vi "数据查询筛选弹框.vi"(8 "error in (no error)":errorcluster caption="错误输入（无错误）", 9 "是否初始化":enum16{"init", "keep"}(ring), 10 "database":string="database1.mdb", 11 "table":string(combo)="CODMn") -> (0 "error out":errorcluster caption="错误输出", 1 "确定输出":bool, 2 "显示项":string[](array[string]), 3 "condition":string)   [LabVIEW 2016]
uses:
  <vilib>/addons/database/Auxilliary.llb/DB Tools DataTypes.ctl
  <vilib>/Utility/miscctls.llb/LVPointTypeDef.ctl
  <vilib>/Utility/sysdir.llb/System Directory Type.ctl
  <vilib>/addons/database/Connection.llb/DB Tools Open Connec (String).vi
  <vilib>/addons/database/Connection.llb/Conn Execute.vi
  <vilib>/addons/database/Recordset.llb/Rec Fetch Recordset Data (R).vi
  <vilib>/addons/database/Recordset.llb/Rec Destroy - Connection.vi
  <userlib>/_OpenG.lib/array/array.llb/Remove Duplicates from 1D Array (String)__ogtk.vi
  <vilib>/addons/database/_DB Variant To Data/Database Variant To Data.xnode
  <vilib>/addons/database/NI_Database_API.lvlib
panel:
  in  "实时分钟小时数据":enum32{"实时数据", "分钟数据", "小时数据"}(radio)
  in  "确定":bool
  out "自定义2single":cluster{"起始范围":string, "截止范围":string}
  out "自定义1single":cluster{"起始范围":string, "截止范围":string}
  out "自定义2筛选条件":string[](array[string])
  out "自定义1筛选条件":string[](array[string])
  in  "标签 2":string="从：\n\n\n至："
  in  "自定义数值结束 2":dbl
  in  "自定义数值起始 2":dbl
  in  "自定义结束时间 2":timestamp
  in  "自定义起始时间 2":timestamp
  in  "自定义 2":T1 caption="自定义"
  in  "组合框 2":string(combo)
  in  "标签":string="从：\n\n\n至："
  in  "自定义数值结束":dbl
  in  "自定义数值起始":dbl
  in  "自定义结束时间":timestamp
  in  "自定义起始时间":timestamp
  in  "自定义":T1
  in  "组合框":string(combo)
  out "type":T2[](array[typedef])
  out "所有测量模式":string[](array[string])
  out "数组":string[](array[string])
  out "columns":string[](array[string])
  in  "测量模式":T3
  in  "退出":bool
  in  "清空":bool
  in  "时间标识输入1":T4 format="%<%Y/%m/%d %H:%M:%S>T"
  in  "时间标识输入2":T4 format="%<%Y/%m/%d %H:%M:%S>T"
  # "实时/分钟/小时数据"
  # "日期"
  # "从："
  # "至："
  # "自定义筛选2"
  # "自定义筛选1"
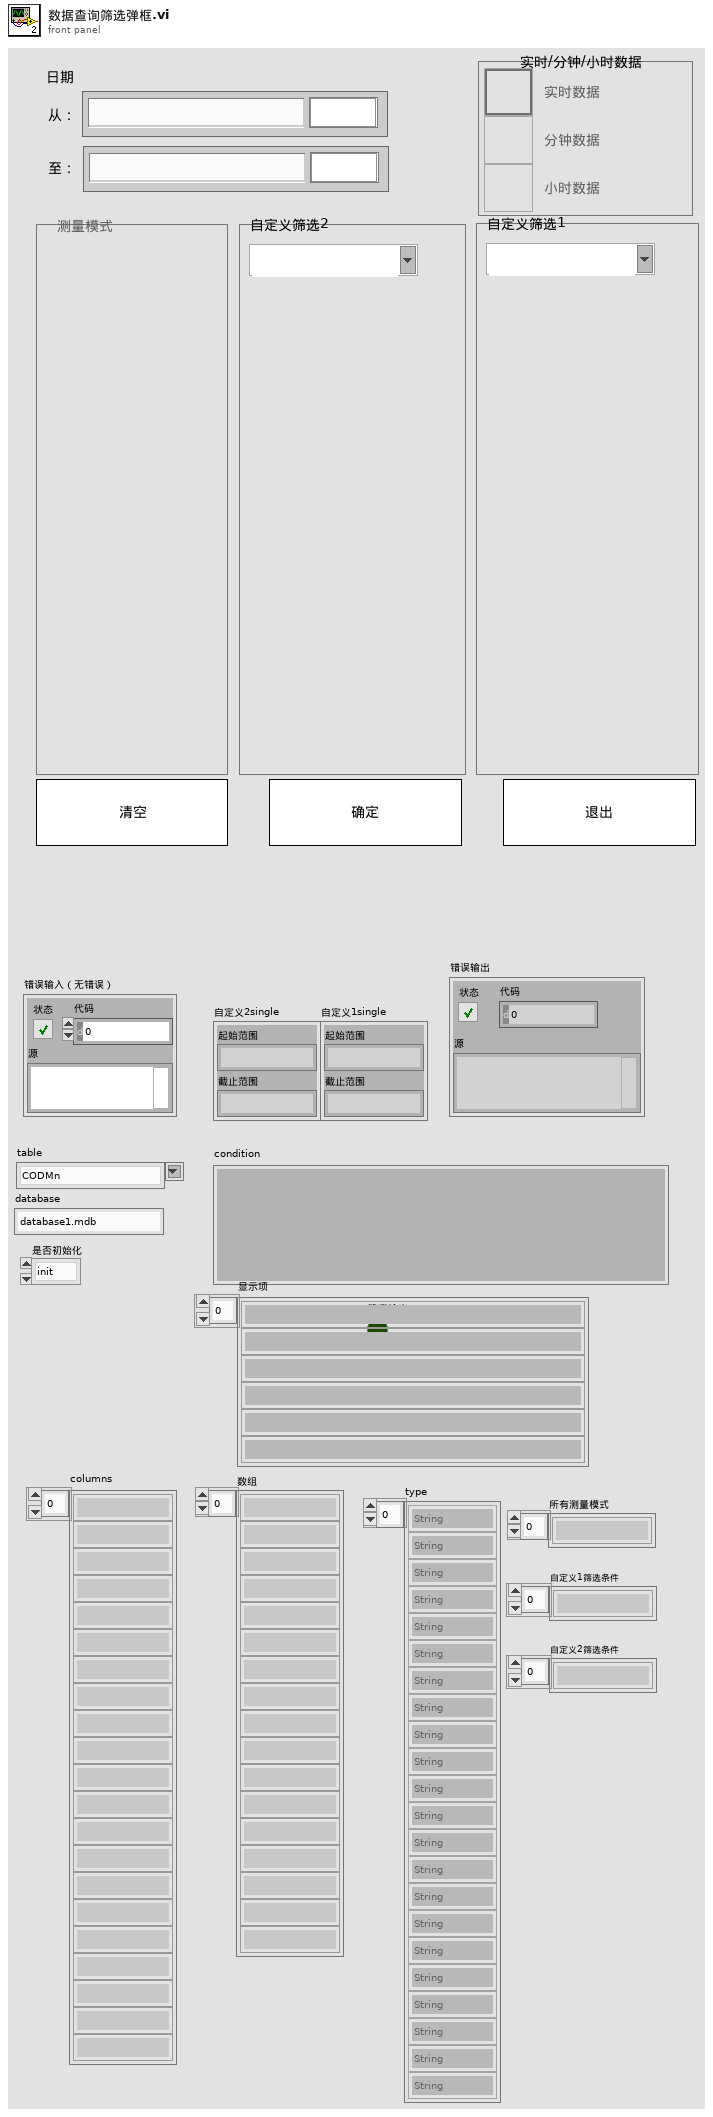
[diagram p1: front panel]
types:
  T1 = cluster{"DSADSA ":bool, "2":bool, "3":bool, "4":bool, "5":bool, "6":bool, "7":bool, "8":bool, "9":bool, "10":bool}
  T2 = typedef "NI_Database_API.lvlib/DB Tools DataTypes.ctl" = enum16{"String", "Long (I32)", "Single (SGL)", "Double (DBL)", "Date/Time", "Binary"}
  T3 = cluster{"水样测试":bool, "标样核查":bool, "零点核查":bool, "跨度核查":bool, "空白测试":bool, "平行样测试":bool, "加标回收":bool, "空白校准":bool, "标样校准":bool, "初始化清洗":bool}
  T4 = typedef "时间标识输入.ctl" = timestamp
  T5 = enum8{"Enabled", "Disabled", "Disabled and Grayed Out"}
  T6 = typedef "LVPointTypeDef.ctl" = cluster{"Horizontal":i16, "Vertical":i16}
  T7 = typedef "System Directory Type.ctl" = i32
  T8 = typedef "NI_Database_API.lvlib/Conn ObjectReference.ctl" = refnum<k1>
  T9 = cluster{"name":string, "database data type":T2, "defined size":i32}[]
  T10 = typedef "NI_Database_API.lvlib/Rec ObjectReference.ctl" = refnum<k1>
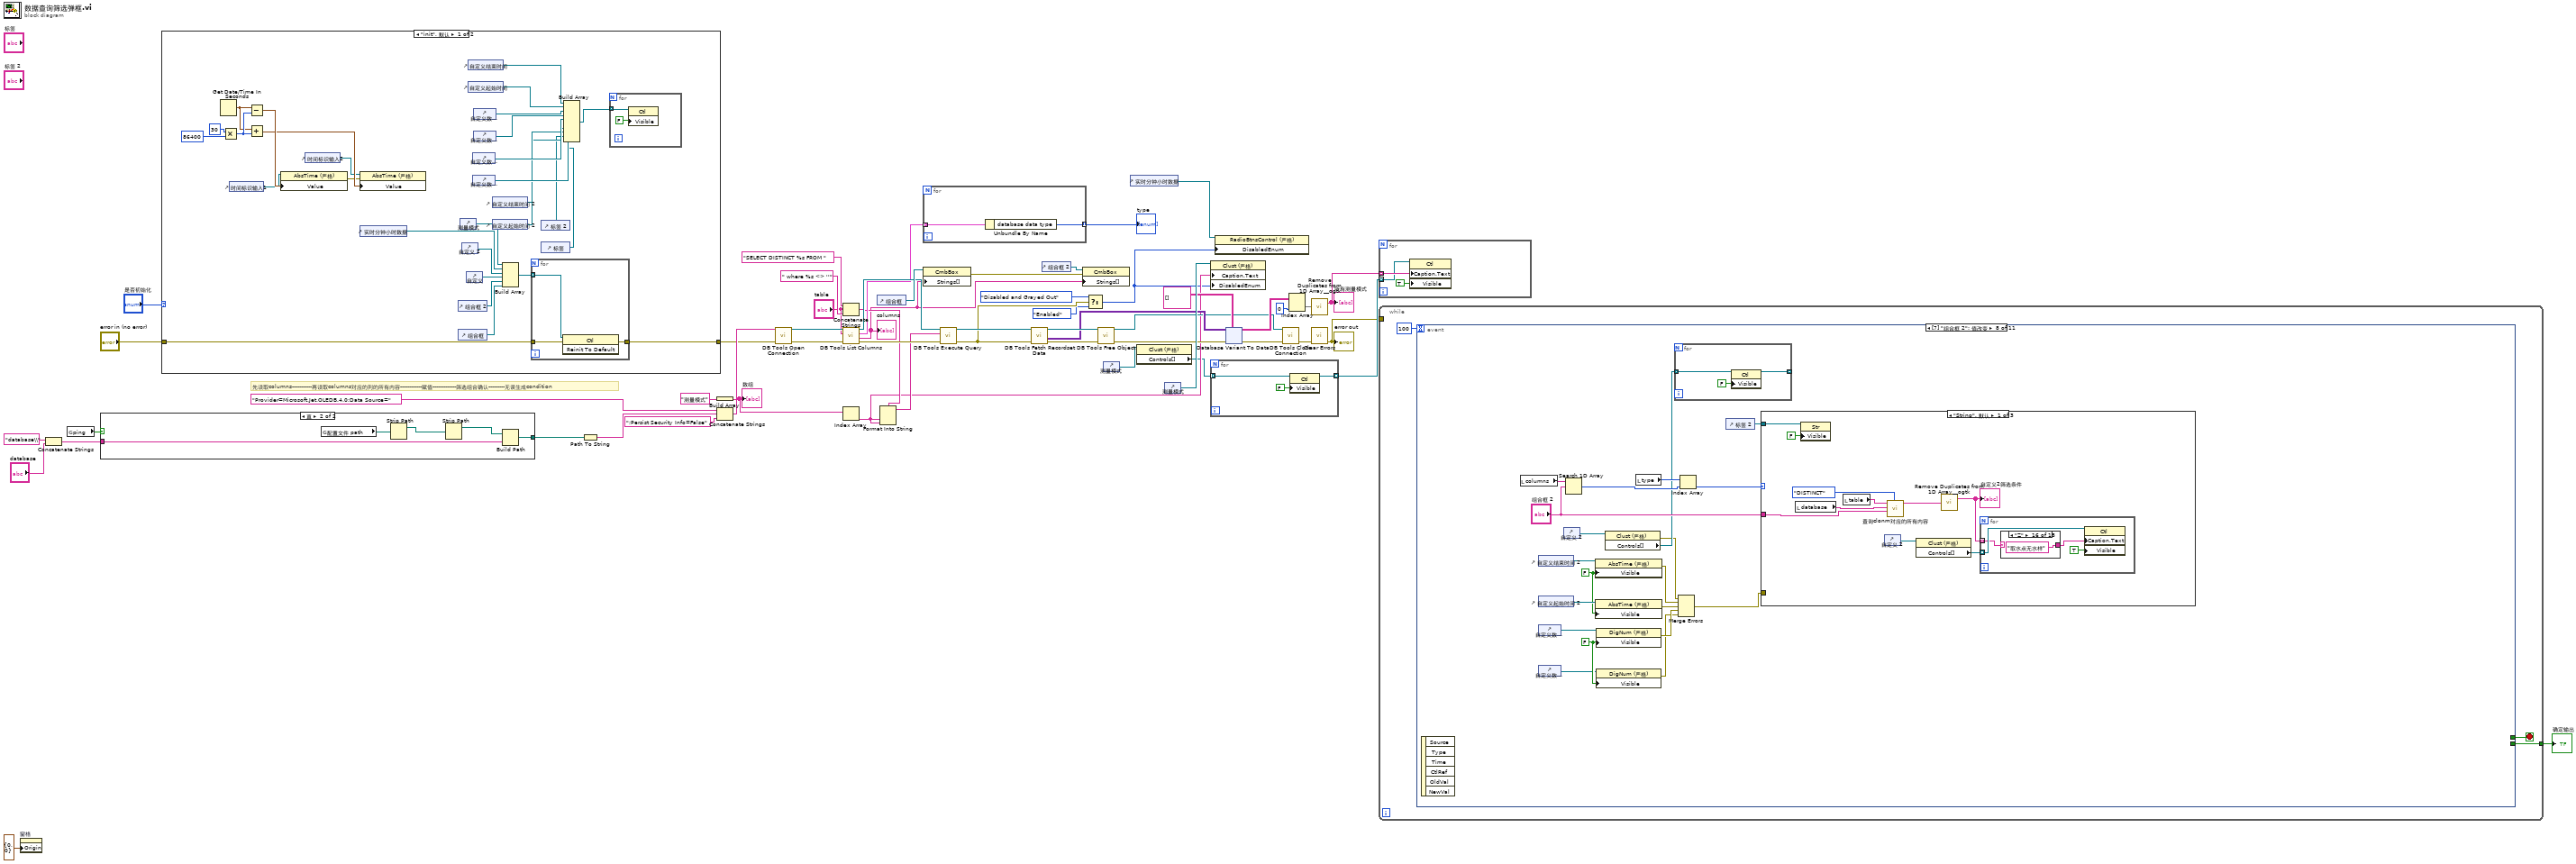
[diagram p0: block diagram]
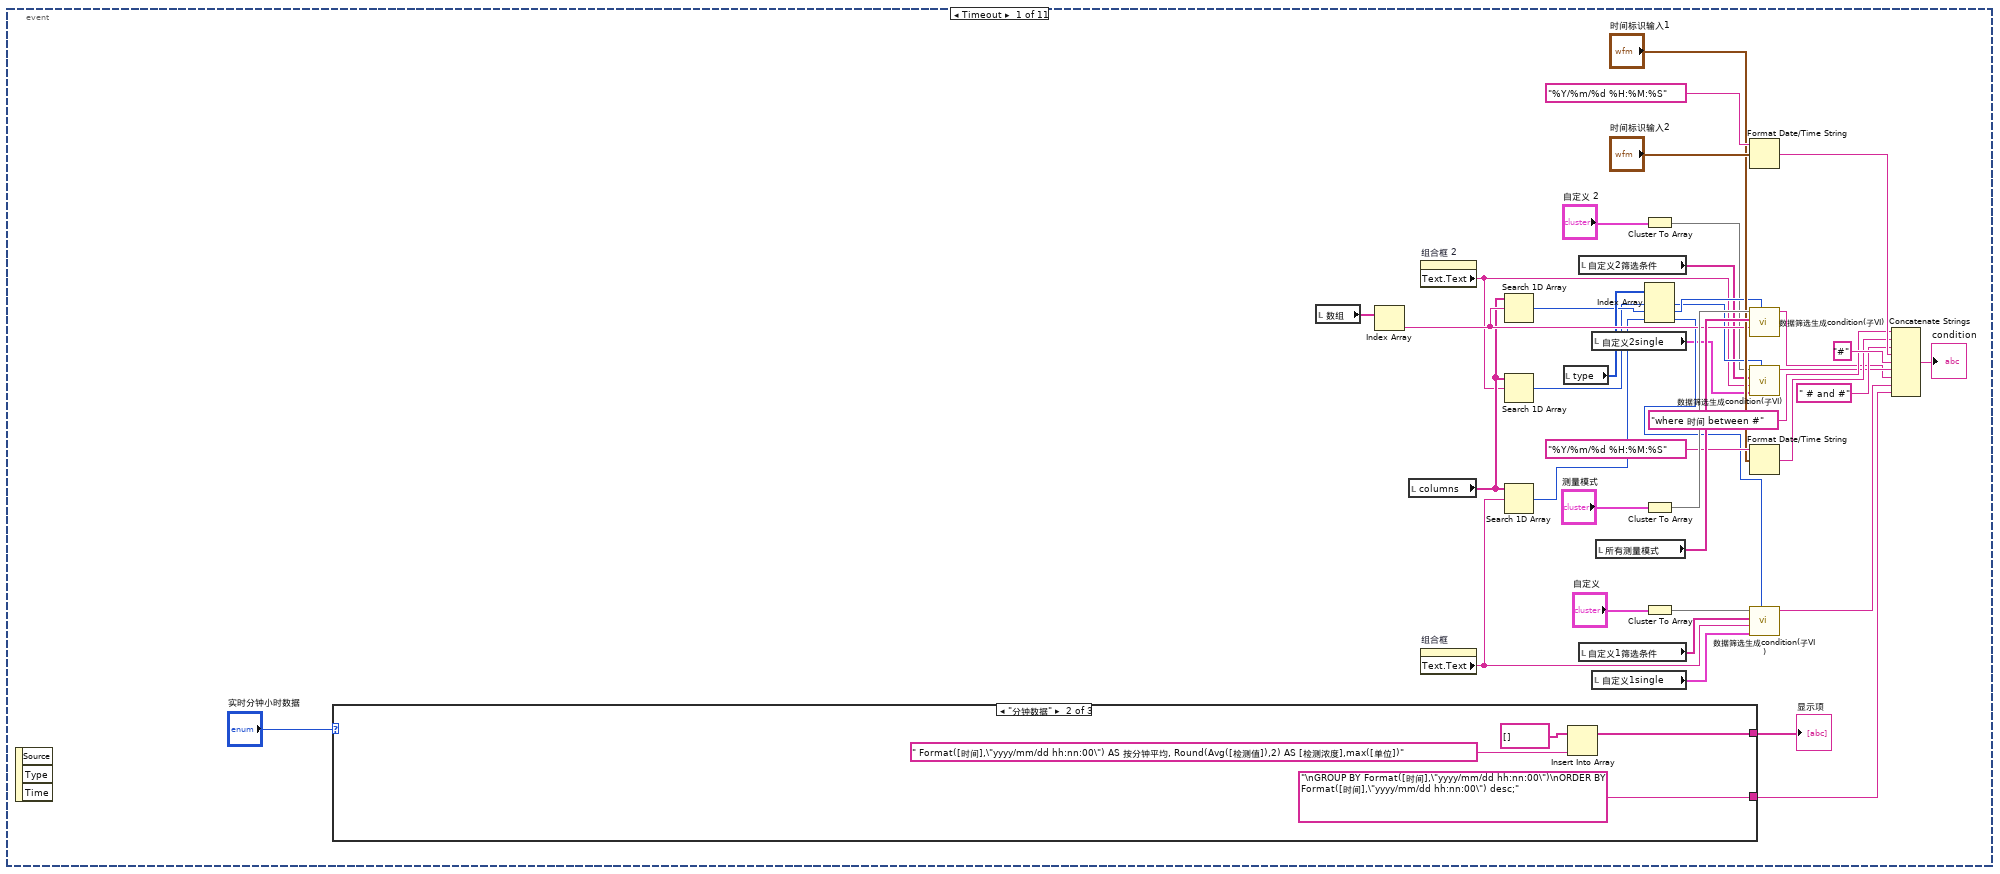
[diagram p3: hidden frame]
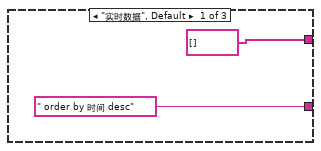
[diagram p4: hidden frame]
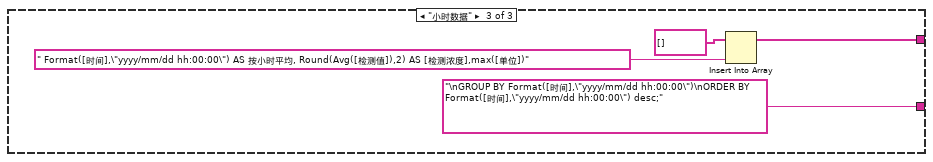
[diagram p5: hidden frame]
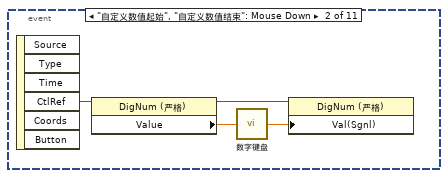
[diagram p6: hidden frame]
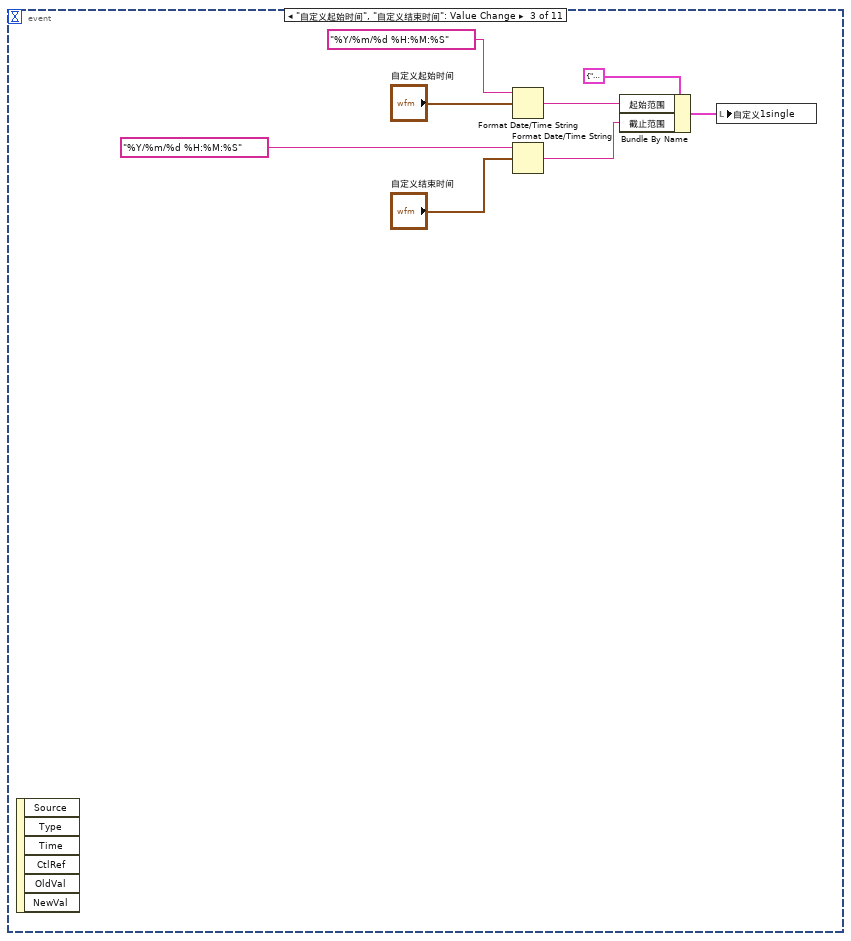
[diagram p7: hidden frame]
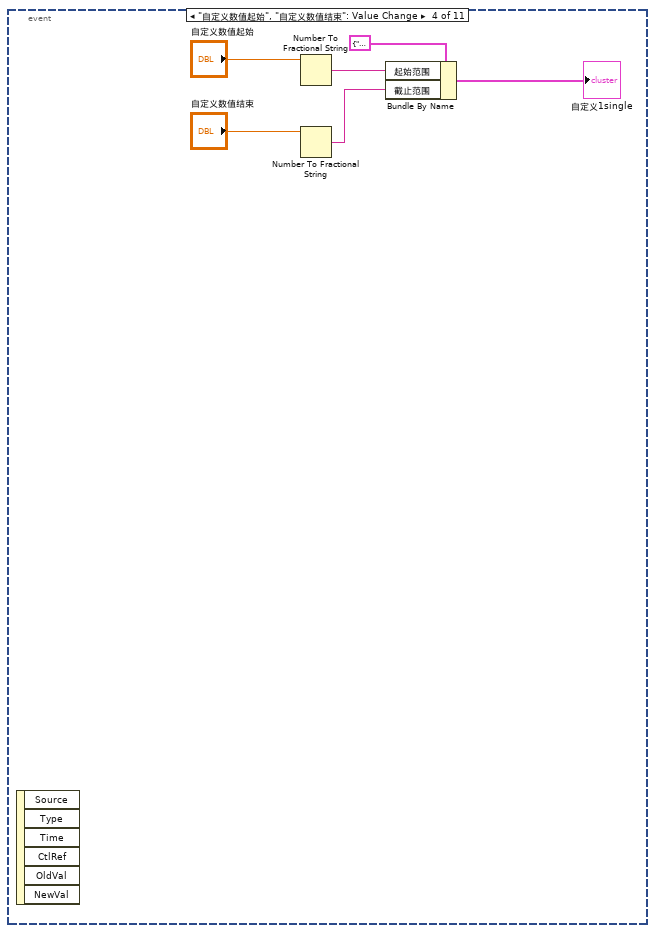
[diagram p8: hidden frame]
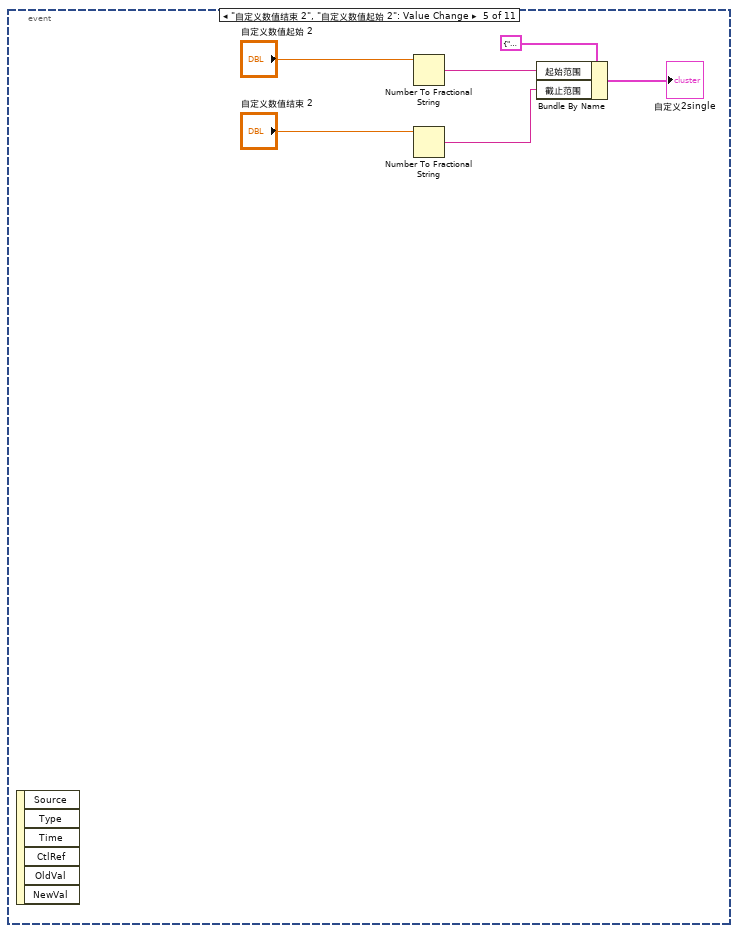
[diagram p9: hidden frame]
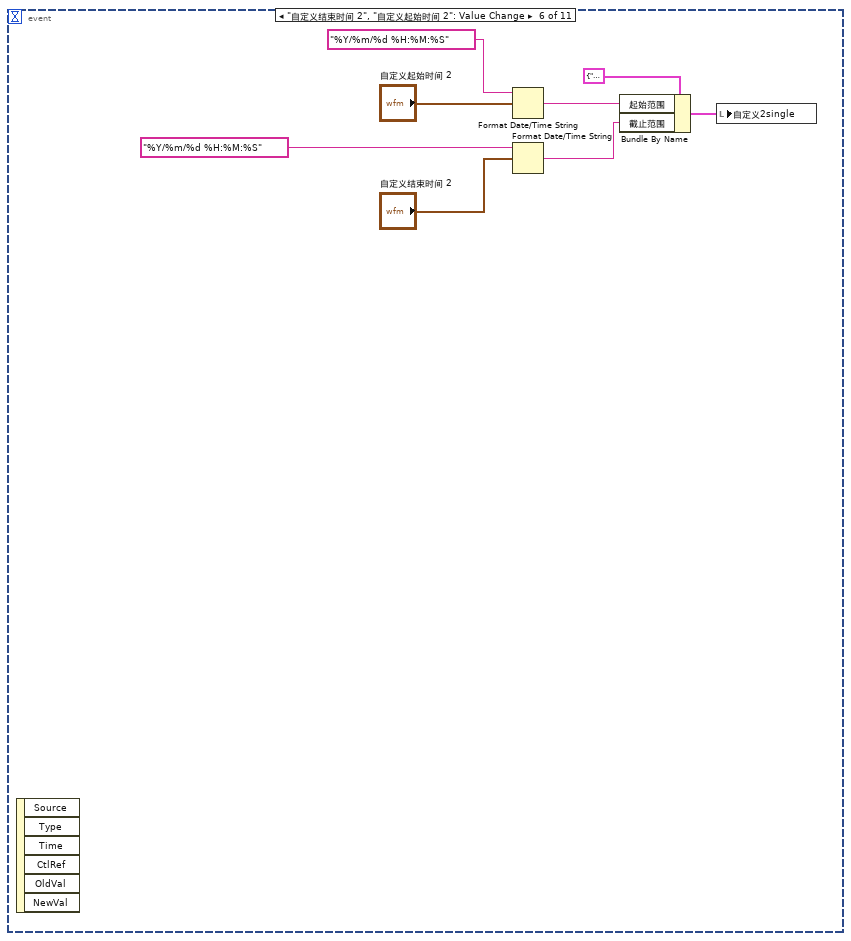
[diagram p10: hidden frame]
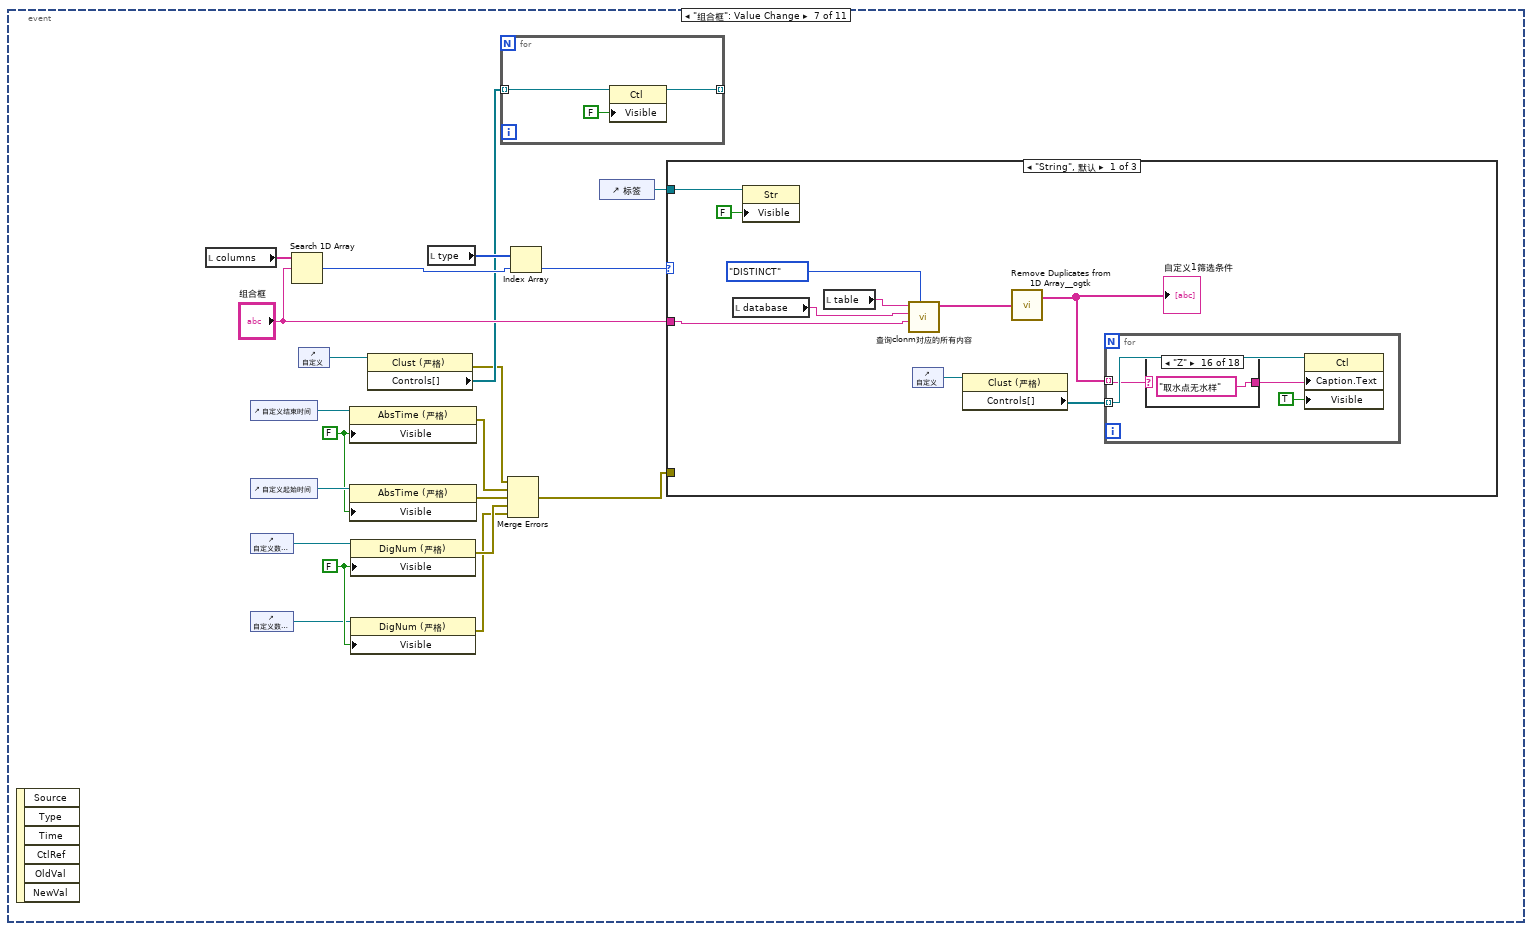
[diagram p11: hidden frame]
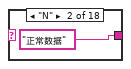
[diagram p13: hidden frame]
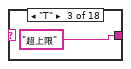
[diagram p14: hidden frame]
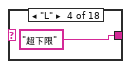
[diagram p15: hidden frame]
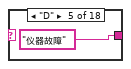
[diagram p16: hidden frame]
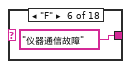
[diagram p17: hidden frame]
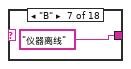
[diagram p18: hidden frame]
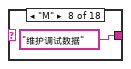
[diagram p19: hidden frame]
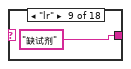
[diagram p20: hidden frame]
diagram:
  # "先读取columns-----------再读取columns对应的列的所有内容------------赋值-------------筛选组合确认---------无误生成condition"
  n1 = property on="窗格" class="Pane"("Origin"=T6 {"Horizontal"=0, "Vertical"=0} ("原点")) -> ()  [unwired: 2 in, 2 out]
  n2 = Concatenate Strings("database\\" ("名称或相对路径"), "database") -> (w47:string)
  n3 = global read "ping全局.vi" "ping"() -> (w48:bool)
  n4 = case shown="真" w48 {
    tunnel: w47 -> [w57 w63]
    tunnel: [w56 w61] -> w46
    frame False {
      w58 = T7 2 items=["用户目录"=0, "用户桌面"=1, "用户文档"=2, "用户应用程序数据"=3, "用户设置"=4, "用户临时目录"=5, "公共文档"=6, "公共应用程序数据"=7, "公共设置"=8, "公共缓存"=13, "系统核心库"=9, "系统安装库"=10, "应用程序文件"=11, "启动盘根目录"=12] ("system directory type")
      n5 = call <vilib>:"Get System Directory.vi"("system directory type"=w58) -> ("system directory"=w59:path)  [unwired: 10 in]
      n6 = Build Path(base path=w59, name or relative path=w57) -> (appended path=w56:path)
    }
    frame True {
      n7 = global read "ping全局.vi" "配置文件 path"() -> (w60:path)
      n8 = Strip Path(path=w60) -> (stripped path=w64:path)  [unwired: 1 out]
      n9 = Strip Path(path=w64) -> (stripped path=w62:path)  [unwired: 1 out]
      n10 = Build Path(base path=w62, name or relative path=w63) -> (appended path=w61:path)
    }
  }
  n11 = case shown="\"init\", 默认" "是否初始化" {
    tunnel: "error in (no error)" -> [w86 w99]
    tunnel: [w85 w99] -> w6
    frame "init", Default {
      n12 = Get Date/Time In Seconds() -> (seconds since 1Jan1904=w76:timestamp)
      n13 = Multiply(x=30, y=86400) -> (x*y=w77:i32)
      n14 = control-ref of="时间标识输入1"() -> (w80:refnum<vi>)
      n15 = Subtract(x=w76, y=w77) -> (x-y=w84:timestamp)
      n16 = Add(x=w76, y=w77) -> (x+y=w83:timestamp)
      n17 = property class="AbsTime (严格)"(reference=w80, "Value"=w84) -> (error out=w82:errorcluster)  [unwired: 1 in, 1 out]
      n18 = control-ref of="时间标识输入2"() -> (w81:refnum<vi>)
      n19 = property class="AbsTime (严格)"(reference=w81, error in=w82, "Value"=w83) -> ()  [unwired: 2 out]
      n20 = control-ref of="实时分钟小时数据"() -> (w91:refnum<vi>)
      n21 = control-ref of="组合框 2"() -> (w93:refnum<vi>)
      n22 = control-ref of="组合框"() -> (w92:refnum<vi>)
      n23 = control-ref of="测量模式"() -> (w87:refnum<vi>)
      n24 = control-ref of="自定义 2"() -> (w90:refnum<vi>)
      n25 = control-ref of="自定义"() -> (w89:refnum<vi>)
      n26 = control-ref of="自定义结束时间"() -> (w75:refnum<vi>)
      n27 = control-ref of="自定义起始时间"() -> (w74:refnum<vi>)
      n28 = control-ref of="自定义数值结束 2"() -> (w71:refnum<vi>)
      n29 = control-ref of="自定义数值起始 2"() -> (w70:refnum<vi>)
      n30 = control-ref of="自定义数值结束"() -> (w73:refnum<vi>)
      n31 = control-ref of="自定义数值起始"() -> (w72:refnum<vi>)
      n32 = control-ref of="自定义结束时间 2"() -> (w68:refnum<vi>)
      n33 = control-ref of="自定义起始时间 2"() -> (w69:refnum<vi>)
      n34 = Build Array(w87, w91, w90, w89, w93, w92) -> (w88:refnum<vi>[])
      n35 = for {
        tunnel: w88 -> [w98] mode=indexing
        tunnel: w86 -> [w97]
        tunnel: [w96] -> w85
        n36 = invoke class="Ctl" method="Reinit To Default"(reference=w98, error in=w97) -> (error out=w96:errorcluster)  [unwired: 1 in, 2 out]
      }
      n37 = control-ref of="标签 2"() -> (w65:refnum<vi>)
      n38 = control-ref of="标签"() -> (w66:refnum<vi>)
      n39 = Build Array(w75, w74, w73, w72, w71, w70, w68, w69, w65, w66) -> (w67:refnum<vi>[])
      n40 = for {
        tunnel: w67 -> [w95] mode=indexing
        n41 = property class="Ctl"(reference=w95, "Visible"=FALSE ("可见")) -> ()  [unwired: 1 in, 2 out]
      }
    }
    frame "keep" {
    }
  }
  n42 = Path To String(path=w46) -> (string=w52:string)
  n43 = Build Array("测量模式" ("Element Data")) -> (w9:string[])
  "数组" <- w9
  n44 = Concatenate Strings("Provider=Microsoft.Jet.OLEDB.4.0;Data Source=", w52, ";Persist Security Info=False") -> (w51:string)
  n45 = call-poly <vilib>:"DB Tools Open Connection.vi"("error in (no error)"=w6, "connection information"=w51) -> ("error out"=w44:errorcluster, "connection reference"=w45:T8)  [unwired: 6 in]
  n46 = Concatenate Strings("SELECT DISTINCT %s FROM " ("字符串"), "table", " where %s <> ''" ("字符串")) -> (w21:string)
  n47 = call <vilib>:"DB Tools List Columns.vi"("error in (no error)"=w44, "table"="table", "connection reference"=w45) -> ("error out"=w38:errorcluster, "columns"=w14:string[], "column information"=w25:T9, "connection reference out"=w26:T8)  [unwired: 1 in]
  "columns" <- w14
  n48 = Index Array(array=w9) -> (element=w19:string)  [unwired: 1 in]
  n49 = control-ref of="组合框"() -> (w27:refnum<vi>)
  n50 = Format Into String(format string=w21, w19, w19) -> (resulting string=w37:string)  [unwired: 2 in, 1 out]
  n51 = for {
    tunnel: w25 -> [w101] mode=indexing
    tunnel: [w100] -> w24 mode=indexing
    n52 = Unbundle By Name(w101) -> ("database data type"=w100:T2)
  }
  "type" <- w24
  n53 = property class="CmbBox"(reference=w27, "Strings[]"=w14) -> (error out=w5:errorcluster)  [unwired: 1 in, 1 out]
  n54 = call-poly <vilib>:"DB Tools Execute Query.vi"("error in (no error)"=w38, "SQL query"=w37, "connection reference"=w26) -> ("error out"=w18:errorcluster, "recordset reference"=w41:T10)  [unwired: 5 in]
  n55 = call-poly <vilib>:"DB Tools Fetch Recordset Data.vi"("error in (no error)"=w18, "recordset reference"=w41) -> ("error out"=w40:errorcluster, "recordset data"=w33:variant[][], "recordset reference out"=w39:T10)  [unwired: 3 in]
  n56 = control-ref of="组合框 2"() -> (w15:refnum<vi>)
  n57 = property class="CmbBox"(reference=w15, error in=w5, "Strings[]"=w14) -> ()  [unwired: 2 out]
  n58 = Select(t=T5."Disabled and Grayed Out" ("禁用"), s=w18, f=T5."Enabled" ("禁用")) -> (s? t:f=w1:T5)
  n59 = call-poly <vilib>:"DB Tools Free Object.vi"("error in (no error)"=w40, "recordset reference"=w39) -> ("error out"=w32:errorcluster, "connection reference"=w31:T8)  [unwired: 8 in]
  n60 = control-ref of="测量模式"() -> (w55:refnum<vi>)
  n61 = control-ref of="实时分钟小时数据"() -> (w2:refnum<vi>)
  n62 = property class="Clust (严格)"(reference=w55) -> ("Controls[]"=w13:refnum<vi>[])  [unwired: 1 in, 2 out]
  n63 = control-ref of="测量模式"() -> (w42:refnum<vi>)
  n64 = property class="Clust (严格)"(reference=w42, "Caption.Text"=w19, "DisabledEnum"=w1) -> ()  [unwired: 1 in, 2 out]
  n65 = for {
    tunnel: w13 -> [w104] mode=indexing
    tunnel: [w102] -> w12 mode=indexing
    n66 = property class="Ctl"(reference=w104, "Visible"=FALSE ("可见")) -> (reference out=w102:refnum<vi>)  [unwired: 1 in, 1 out]
  }
  n67 = property class="RadioBtnsControl (严格)"(reference=w2, "DisabledEnum"=w1) -> ()  [unwired: 1 in, 2 out]
  n68 = xnode "Database Variant To Data"("database variant"=w33, "error in (no error)"=w32, "type"=string[][] []) -> ("data"=w34:string[][], "error out"=w35:errorcluster)
  n69 = call <vilib>:"DB Tools Close Connection.vi"("error in (no error)"=w35, "connection reference"=w31) -> ("error out"=w8:errorcluster)  [unwired: 5 in]
  n70 = Index Array(array=w34, index (col)=0 ("禁用的索引 (列)")) -> (element=w29:string[])  [unwired: 1 in]
  n71 = call-poly <userlib>:"Remove Duplicates from 1D Array__ogtk.vi"("Input Array"=w29) -> ("Output Array"=w11:string[])  [unwired: 1 out]
  "所有测量模式" <- w11
  n72 = call <vilib>:"Clear Errors.vi"("error in (no error)"=w8) -> ("error out"=w3:errorcluster)  [unwired: 5 in, 1 out]
  "error out" <- w3
  n73 = for {
    tunnel: w11 -> [w107] mode=indexing
    tunnel: w12 -> [w105] mode=indexing
    n74 = property class="Ctl"(reference=w105, "Caption.Text"=w107, "Visible"=TRUE ("可见")) -> ()  [unwired: 1 in, 2 out]
  }
  n75 = while {
    tunnel: [w108] -> w10
    tunnel: w3 -> [_]
    stop <- w110 stop-if-true
    n76 = event shown="[7] \"组合框 2\": 值改变" {
      selector: _ -> [_ _ _ _ _ _ _ _ _ _ _]
      dyn-events: _ -> [_ _ _ _ _ _ _ _ _ _ _]
      timeout: 100 -> [_ _ _ _ _ _ _ _ _ _ _]
      tunnel: [_ _ _ _ _ _ _ _ _ w388 TRUE] -> w110
      tunnel: [_ _ _ _ _ _ _ _ _ w388 _] -> w108
      event Timeout {
        n77 = event-data() -> ()  [unwired: 1 in, 3 out]
        n78 = case shown="\"分钟数据\"" "实时分钟小时数据" {
          tunnel: [string[] [] ("显示项") w152 w156] -> w111
          tunnel: [" order by 时间 desc" ("字符串") "\nGROUP BY Format([时间],\"yyyy/mm/dd hh:nn:00\")\nORDER BY Format([时间],\"yyyy/mm/dd hh:nn:00\") desc;" ("字符串") "\nGROUP BY Format([时间],\"yyyy/mm/dd hh:00:00\")\nORDER BY Format([时间],\"yyyy/mm/dd hh:00:00\") desc;" ("字符串")] -> w112
          frame "实时数据", Default {
          }
          frame "分钟数据" {
            n79 = Insert Into Array(array=string[] [] ("显示项"), new element=" Format([时间],\"yyyy/mm/dd hh:nn:00\") AS 按分钟平均, Round(Avg([检测值]),2) AS [检测浓度],max([单位])" ("新元素/子数组")) -> (w152:string[])  [unwired: 1 in]
          }
          frame "小时数据" {
            n80 = Insert Into Array(array=string[] [] ("显示项"), new element=" Format([时间],\"yyyy/mm/dd hh:00:00\") AS 按小时平均, Round(Avg([检测值]),2) AS [检测浓度],max([单位])" ("新元素/子数组")) -> (w156:string[])  [unwired: 1 in]
          }
        }
        "显示项" <- w111
        n81 = local read "数组"() -> (w149:string[])
        n82 = Index Array(array=w149) -> (element=w135:string)  [unwired: 1 in]
        n83 = local read "columns"() -> (w129:string[])
        n84 = property on="组合框 2" class="CmbBox"() -> ("Text.Text"=w120:string)  [unwired: 2 in, 2 out]
        n85 = property on="组合框" class="CmbBox"() -> ("Text.Text"=w119:string)  [unwired: 2 in, 2 out]
        n86 = Search 1D Array(1D array=w129, element=w135) -> (index of element=w133:i32)  [unwired: 1 in]
        n87 = Search 1D Array(1D array=w129, element=w120) -> (index of element=w128:i32)  [unwired: 1 in]
        n88 = Search 1D Array(1D array=w129, element=w119) -> (index of element=w131:i32)  [unwired: 1 in]
        n89 = local read "type"() -> (w134:T2[])
        n90 = local read "自定义2筛选条件"() -> (w117:string[])
        n91 = local read "自定义1筛选条件"() -> (w118:string[])
        n92 = local read "自定义2single"() -> (w115:cluster{"起始范围":string, "截止范围":string})
        n93 = local read "自定义1single"() -> (w114:cluster{"起始范围":string, "截止范围":string})
        n94 = local read "所有测量模式"() -> (w148:string[])
        n95 = Cluster To Array(cluster="自定义 2") -> (array=w126:bool[])
        n96 = Index Array(array=w134, index #1=w128, index #2=w133, index #3=w131) -> (element #1=w127:T2, element #2=w132:T2, element #3=w130:T2)
        n97 = Cluster To Array(cluster="测量模式") -> (array=w147:bool[])
        n98 = Cluster To Array(cluster="自定义") -> (array=w116:bool[])
        n99 = Format Date/Time String(time format string (%c)="%Y/%m/%d %H:%M:%S" ("时间格式字符串(%c)"), seconds (now)="时间标识输入2") -> (date/time string=w144:string)  [unwired: 1 in]
        n100 = call "数据筛选生成condition(子VI).vi"("database data type"=w132, "段名"=w135, "筛选内容"=w148, "簇转数组"=w147) -> ("condition"=w124:string)  [unwired: 7 in]
        n101 = call "数据筛选生成condition(子VI).vi"("database data type"=w127, "Single"=w115, "段名"=w120, "筛选内容"=w117, "簇转数组"=w126) -> ("condition"=w125:string)  [unwired: 6 in]
        n102 = Format Date/Time String(time format string (%c)="%Y/%m/%d %H:%M:%S" ("时间格式字符串(%c)"), seconds (now)="时间标识输入1") -> (date/time string=w142:string)  [unwired: 1 in]
        n103 = call "数据筛选生成condition(子VI).vi"("database data type"=w130, "Single"=w114, "段名"=w119, "筛选内容"=w118, "簇转数组"=w116) -> ("condition"=w123:string)  [unwired: 6 in]
        n104 = Concatenate Strings("where 时间 between #", w142, " # and #" ("condition"), w144, "#" ("condition"), w125, w124, w123, w112) -> (→"condition":string)
      }
      event "自定义数值起始", "自定义数值结束": Mouse Down {
        n105 = event-data() -> ("CtlRef"=w163:refnum<vi>)  [unwired: 1 in, 5 out]
        n106 = property class="DigNum (严格)"(reference=w163) -> (reference out=w161:refnum<vi>, "Value"=w162:dbl)  [unwired: 1 in, 1 out]
        n107 = call "数字键盘.vi"("OldNumber"=w162) -> ("NewNumber"=w160:sgl)
        n108 = property class="DigNum (严格)"(reference=w161, "Val(Sgnl)"=w160) -> ()  [unwired: 1 in, 2 out]
      }
      event "自定义起始时间", "自定义结束时间": Value Change {
        n109 = event-data() -> ()  [unwired: 1 in, 6 out]
        n110 = Format Date/Time String(time format string (%c)="%Y/%m/%d %H:%M:%S" ("时间格式字符串(%c)"), seconds (now)="自定义起始时间") -> (date/time string=w170:string)  [unwired: 1 in]
        n111 = Format Date/Time String(time format string (%c)="%Y/%m/%d %H:%M:%S" ("时间格式字符串(%c)"), seconds (now)="自定义结束时间") -> (date/time string=w171:string)  [unwired: 1 in]
        n112 = Bundle By Name(cluster=cluster{"起始范围":string, "截止范围":string} {"起始范围"="2", "截止范围"="5"} ("Single"), "起始范围"=w170, "截止范围"=w171) -> (w164:cluster{"起始范围":string, "截止范围":string})
        n113 = local write "自定义1single"(w164) -> ()
      }
      event "自定义数值起始", "自定义数值结束": Value Change {
        n114 = event-data() -> ()  [unwired: 1 in, 6 out]
        n115 = Number To Fractional String(number="自定义数值起始") -> (F-format string=w176:string)  [unwired: 3 in]
        n116 = Number To Fractional String(number="自定义数值结束") -> (F-format string=w177:string)  [unwired: 3 in]
        n117 = Bundle By Name(cluster=cluster{"起始范围":string, "截止范围":string} {"起始范围"="2", "截止范围"="5"} ("Single"), "起始范围"=w176, "截止范围"=w177) -> (→"自定义1single":cluster{"起始范围":string, "截止范围":string})
      }
      event "自定义数值结束 2", "自定义数值起始 2": Value Change {
        n118 = event-data() -> ()  [unwired: 1 in, 6 out]
        n119 = Number To Fractional String(number="自定义数值起始 2") -> (F-format string=w180:string)  [unwired: 3 in]
        n120 = Number To Fractional String(number="自定义数值结束 2") -> (F-format string=w179:string)  [unwired: 3 in]
        n121 = Bundle By Name(cluster=cluster{"起始范围":string, "截止范围":string} {"起始范围"="2", "截止范围"="5"} ("Single"), "起始范围"=w180, "截止范围"=w179) -> (→"自定义2single":cluster{"起始范围":string, "截止范围":string})
      }
      event "自定义结束时间 2", "自定义起始时间 2": Value Change {
        n122 = event-data() -> ()  [unwired: 1 in, 6 out]
        n123 = Format Date/Time String(time format string (%c)="%Y/%m/%d %H:%M:%S" ("时间格式字符串(%c)"), seconds (now)="自定义起始时间 2") -> (date/time string=w189:string)  [unwired: 1 in]
        n124 = Format Date/Time String(time format string (%c)="%Y/%m/%d %H:%M:%S" ("时间格式字符串(%c)"), seconds (now)="自定义结束时间 2") -> (date/time string=w190:string)  [unwired: 1 in]
        n125 = Bundle By Name(cluster=cluster{"起始范围":string, "截止范围":string} {"起始范围"="2", "截止范围"="5"} ("Single"), "起始范围"=w189, "截止范围"=w190) -> (w191:cluster{"起始范围":string, "截止范围":string})
        n126 = local write "自定义2single"(w191) -> ()
      }
      event "组合框": Value Change {
        w202 = FALSE ("可见")
        w192 = FALSE ("可见")
        n127 = event-data() -> ()  [unwired: 1 in, 6 out]
        n128 = local read "columns"() -> (w209:string[])
        n129 = control-ref of="自定义结束时间"() -> (w204:refnum<vi>)
        n130 = control-ref of="自定义起始时间"() -> (w203:refnum<vi>)
        n131 = control-ref of="自定义数值结束"() -> (w201:refnum<vi>)
        n132 = control-ref of="自定义数值起始"() -> (w194:refnum<vi>)
        n133 = Search 1D Array(1D array=w209, element="组合框") -> (index of element=w211:i32)  [unwired: 1 in]
        n134 = control-ref of="自定义"() -> (w206:refnum<vi>)
        n135 = property class="AbsTime (严格)"(reference=w204, "Visible"=w192) -> (error out=w199:errorcluster)  [unwired: 1 in, 1 out]
        n136 = property class="AbsTime (严格)"(reference=w203, "Visible"=w192) -> (error out=w198:errorcluster)  [unwired: 1 in, 1 out]
        n137 = property class="DigNum (严格)"(reference=w201, "Visible"=w202) -> (error out=w197:errorcluster)  [unwired: 1 in, 1 out]
        n138 = property class="DigNum (严格)"(reference=w194, "Visible"=w202) -> (error out=w196:errorcluster)  [unwired: 1 in, 1 out]
        n139 = property class="Clust (严格)"(reference=w206) -> (error out=w200:errorcluster, "Controls[]"=w205:refnum<vi>[])  [unwired: 1 in, 1 out]
        n140 = local read "type"() -> (w210:T2[])
        n141 = for {
          tunnel: w205 -> [w214] mode=indexing
          tunnel: [w212] -> _ mode=indexing
          n142 = property class="Ctl"(reference=w214, "Visible"=FALSE ("可见")) -> (reference out=w212:refnum<vi>)  [unwired: 1 in, 1 out]
        }
        n143 = Merge Errors(w200, w199, w198, w197, w196) -> (w195:errorcluster)
        n144 = Index Array(array=w210, index=w211) -> (element=w207:T2)
        n145 = control-ref of="标签"() -> (w193:refnum<vi>)
        n146 = case shown="\"String\", 默认" w207 {
          tunnel: "组合框" -> [w222 w254 w275]
          tunnel: w195 -> [_ _ _]
          tunnel: w193 -> [w217 w260 w280]
          frame "String", Default {
            n147 = local read "database"() -> (w223:string)
            n148 = property class="Str"(reference=w217, "Visible"=FALSE ("可见")) -> ()  [unwired: 1 in, 2 out]
            n149 = local read "table"() -> (w224:string)
            n150 = call "查询clonm对应的所有内容.vi"("条件"=enum16{"DISTINCT", "MIN", "MAX"}."DISTINCT", "组合框"=w222, "database"=w223, "table"=w224) -> ("输出数组"=w221:string[])  [unwired: 6 in, 1 out]
            n151 = control-ref of="自定义"() -> (w219:refnum<vi>)
            n152 = property class="Clust (严格)"(reference=w219) -> ("Controls[]"=w218:refnum<vi>[])  [unwired: 1 in, 2 out]
            n153 = call-poly <userlib>:"Remove Duplicates from 1D Array__ogtk.vi"("Input Array"=w221) -> ("Output Array"=w220:string[])  [unwired: 1 out]
            "自定义1筛选条件" <- w220
            n154 = for {
              tunnel: w220 -> [w225] mode=indexing
              tunnel: w218 -> [w227] mode=indexing
              n155 = case shown="\"Z\"" w225 {
                selector: w225 -> [w229 _ _ _ _ _ _ _ _ _ _ _ _ _ _ _ _ _]
                tunnel: [w229 "正常数据" "超上限" "超下限" "仪器故障" "仪器通信故障" "仪器离线" "维护调试数据" "缺试剂" "缺纯水" "缺水样" "缺标液" "加标回收" "平行样测试" "电源故障" "取水点无水样" "手工输入数据" "手动测试数据"] -> w226
                frame Default {
                }
                frame "N" {
                }
                frame "T" {
                }
                frame "L" {
                }
                frame "D" {
                }
                frame "F" {
                }
                frame "B" {
                }
                frame "M" {
                }
                frame "lr" {
                }
                frame "lp" {
                }
                frame "lw" {
                }
                frame "ls" {
                }
                frame "ra" {
                }
                frame "pt" {
                }
                frame "P" {
                }
                frame "Z" {
                }
                frame "S" {
                }
                frame "hd" {
                }
              }
              n156 = property class="Ctl"(reference=w227, "Caption.Text"=w226, "Visible"=TRUE ("可见")) -> ()  [unwired: 1 in, 2 out]
            }
          }
          frame "Long (I32)".."Double (DBL)" {
            w262 = TRUE ("可见")
            n157 = local read "database"() -> (w255:string)
            n158 = property class="Str"(reference=w260, "Visible"=TRUE ("可见")) -> ()  [unwired: 1 in, 2 out]
            n159 = local read "table"() -> (w256:string)
            n160 = call "查询clonm对应的所有内容.vi"("条件"=enum16{"DISTINCT", "MIN", "MAX"}."MAX", "组合框"=w254, "database"=w255, "table"=w256) -> ("输出数组"=w253:string[])  [unwired: 6 in, 1 out]
            n161 = call "查询clonm对应的所有内容.vi"("条件"=enum16{"DISTINCT", "MIN", "MAX"}."MIN", "组合框"=w254, "database"=w255, "table"=w256) -> ("输出数组"=w258:string[])  [unwired: 6 in, 1 out]
            n162 = Index Array(array=w253) -> (element=w248:string)  [unwired: 1 in]
            n163 = Index Array(array=w258) -> (element=w247:string)  [unwired: 1 in]
            n164 = control-ref of="自定义数值结束"() -> (w263:refnum<vi>)
            n165 = control-ref of="自定义数值起始"() -> (w264:refnum<vi>)
            n166 = Fract/Exp String To Number(string=w248) -> (number=w251:dbl)  [unwired: 3 in, 1 out]
            n167 = Fract/Exp String To Number(string=w247) -> (number=w252:dbl)  [unwired: 3 in, 1 out]
            n168 = Bundle By Name(cluster=cluster{"起始范围":string, "截止范围":string} {"起始范围"="2", "截止范围"="5"} ("Single"), "起始范围"=w247, "截止范围"=w248) -> (w249:cluster{"起始范围":string, "截止范围":string})
            n169 = property class="DigNum (严格)"(reference=w263, "Visible"=w262, "Value"=w251) -> ()  [unwired: 1 in, 2 out]
            n170 = property class="DigNum (严格)"(reference=w264, "Visible"=w262, "Value"=w252) -> ()  [unwired: 1 in, 2 out]
            n171 = local write "自定义1single"(w249) -> ()
          }
          frame "Date/Time" {
            n172 = local read "database"() -> (w276:string)
            n173 = property class="Str"(reference=w280, "Visible"=TRUE ("可见")) -> ()  [unwired: 1 in, 2 out]
            n174 = local read "table"() -> (w277:string)
            n175 = call "查询clonm对应的所有内容.vi"("条件"=enum16{"DISTINCT", "MIN", "MAX"}."MAX", "组合框"=w275, "database"=w276, "table"=w277) -> ("输出数组"=w274:string[])  [unwired: 6 in, 1 out]
            n176 = call "查询clonm对应的所有内容.vi"("条件"=enum16{"DISTINCT", "MIN", "MAX"}."MIN", "组合框"=w275, "database"=w276, "table"=w277) -> ("输出数组"=w269:string[])  [unwired: 6 in, 1 out]
            n177 = Index Array(array=w274) -> (element=w268:string)  [unwired: 1 in]
            n178 = Index Array(array=w269) -> (element=w266:string)  [unwired: 1 in]
            n179 = call "格式日期时间字符串.vi"("data[0]"=w268) -> ("日期/时间字符串"=w267:string)  [unwired: 10 in]
            n180 = call "格式日期时间字符串.vi"("data[0]"=w266) -> ("日期/时间字符串"=w265:string)  [unwired: 10 in]
            n181 = control-ref of="自定义起始时间"() -> (w282:refnum<vi>)
            n182 = control-ref of="自定义结束时间"() -> (w283:refnum<vi>)
            n183 = call "日期字符串格式至时间格式转换(子VI).vi"("data[0]"=w267) -> ("time stamp"=w272:timestamp)  [unwired: 10 in]
            n184 = call "日期字符串格式至时间格式转换(子VI).vi"("data[0]"=w265) -> ("time stamp"=w273:timestamp)  [unwired: 10 in]
            n185 = Bundle By Name(cluster=cluster{"起始范围":string, "截止范围":string} {"起始范围"="2", "截止范围"="5"} ("Single"), "起始范围"=w265, "截止范围"=w267) -> (w270:cluster{"起始范围":string, "截止范围":string})
            n186 = property class="AbsTime (严格)"(reference=w282, "Visible"=TRUE ("可见"), "Value"=w273) -> ()  [unwired: 1 in, 2 out]
            n187 = local write "自定义1single"(w270) -> ()
            n188 = property class="AbsTime (严格)"(reference=w283, "Visible"=TRUE ("可见"), "Value"=w272) -> ()  [unwired: 1 in, 2 out]
          }
        }
      }
      event "组合框 2": Value Change {
        w296 = FALSE ("可见")
        w286 = FALSE ("可见")
        n189 = event-data() -> ()  [unwired: 1 in, 6 out]
        n190 = local read "columns"() -> (w302:string[])
        n191 = control-ref of="自定义结束时间 2"() -> (w298:refnum<vi>)
        n192 = control-ref of="自定义起始时间 2"() -> (w297:refnum<vi>)
        n193 = control-ref of="自定义数值结束 2"() -> (w295:refnum<vi>)
        n194 = control-ref of="自定义数值起始 2"() -> (w288:refnum<vi>)
        n195 = control-ref of="自定义 2"() -> (w300:refnum<vi>)
        n196 = Search 1D Array(1D array=w302, element="组合框 2") -> (index of element=w304:i32)  [unwired: 1 in]
        n197 = property class="AbsTime (严格)"(reference=w298, "Visible"=w286) -> (error out=w293:errorcluster)  [unwired: 1 in, 1 out]
        n198 = property class="AbsTime (严格)"(reference=w297, "Visible"=w286) -> (error out=w292:errorcluster)  [unwired: 1 in, 1 out]
        n199 = property class="DigNum (严格)"(reference=w295, "Visible"=w296) -> (error out=w291:errorcluster)  [unwired: 1 in, 1 out]
        n200 = property class="DigNum (严格)"(reference=w288, "Visible"=w296) -> (error out=w290:errorcluster)  [unwired: 1 in, 1 out]
        n201 = property class="Clust (严格)"(reference=w300) -> (error out=w294:errorcluster, "Controls[]"=w299:refnum<vi>[])  [unwired: 1 in, 1 out]
        n202 = local read "type"() -> (w303:T2[])
        n203 = for {
          tunnel: w299 -> [w308] mode=indexing
          tunnel: [w306] -> _ mode=indexing
          n204 = property class="Ctl"(reference=w308, "Visible"=FALSE ("可见")) -> (reference out=w306:refnum<vi>)  [unwired: 1 in, 1 out]
        }
        n205 = Merge Errors(w294, w293, w292, w291, w290) -> (w289:errorcluster)
        n206 = Index Array(array=w303, index=w304) -> (element=w301:T2)
        n207 = control-ref of="标签 2"() -> (w287:refnum<vi>)
        n208 = case shown="\"String\", 默认" w301 {
          tunnel: "组合框 2" -> [w316 w349 w367]
          tunnel: w289 -> [_ _ _]
          tunnel: w287 -> [w312 w354 w374]
          frame "String", Default {
            n209 = local read "database"() -> (w317:string)
            n210 = property class="Str"(reference=w312, "Visible"=FALSE ("可见")) -> ()  [unwired: 1 in, 2 out]
            n211 = local read "table"() -> (w318:string)
            n212 = control-ref of="自定义 2"() -> (w314:refnum<vi>)
            n213 = call "查询clonm对应的所有内容.vi"("条件"=enum16{"DISTINCT", "MIN", "MAX"}."DISTINCT", "组合框"=w316, "database"=w317, "table"=w318) -> ("输出数组"=w315:string[])  [unwired: 6 in, 1 out]
            n214 = property class="Clust (严格)"(reference=w314) -> ("Controls[]"=w313:refnum<vi>[])  [unwired: 1 in, 2 out]
            n215 = call-poly <userlib>:"Remove Duplicates from 1D Array__ogtk.vi"("Input Array"=w315) -> ("Output Array"=w309:string[])  [unwired: 1 out]
            "自定义2筛选条件" <- w309
            n216 = for {
              tunnel: w309 -> [w320] mode=indexing
              tunnel: w313 -> [w321] mode=indexing
              n217 = case shown="\"Z\"" w320 {
                selector: w320 -> [w323 _ _ _ _ _ _ _ _ _ _ _ _ _ _ _ _ _]
                tunnel: [w323 "正常数据" "超上限" "超下限" "仪器故障" "仪器通信故障" "仪器离线" "维护调试数据" "缺试剂" "缺纯水" "缺水样" "缺标液" "加标回收" "平行样测试" "电源故障" "取水点无水样" "手工输入数据" "手动测试数据"] -> w319
                frame Default {
                }
                frame "N" {
                }
                frame "T" {
                }
                frame "L" {
                }
                frame "D" {
                }
                frame "F" {
                }
                frame "B" {
                }
                frame "M" {
                }
                frame "lr" {
                }
                frame "lp" {
                }
                frame "lw" {
                }
                frame "ls" {
                }
                frame "ra" {
                }
                frame "pt" {
                }
                frame "P" {
                }
                frame "Z" {
                }
                frame "S" {
                }
                frame "hd" {
                }
              }
              n218 = property class="Ctl"(reference=w321, "Caption.Text"=w319, "Visible"=TRUE ("可见")) -> ()  [unwired: 1 in, 2 out]
            }
          }
          frame "Long (I32)".."Double (DBL)" {
            w356 = TRUE ("可见")
            n219 = local read "database"() -> (w350:string)
            n220 = property class="Str"(reference=w354, "Visible"=TRUE ("可见")) -> ()  [unwired: 1 in, 2 out]
            n221 = local read "table"() -> (w351:string)
            n222 = call "查询clonm对应的所有内容.vi"("条件"=enum16{"DISTINCT", "MIN", "MAX"}."MAX", "组合框"=w349, "database"=w350, "table"=w351) -> ("输出数组"=w348:string[])  [unwired: 6 in, 1 out]
            n223 = call "查询clonm对应的所有内容.vi"("条件"=enum16{"DISTINCT", "MIN", "MAX"}."MIN", "组合框"=w349, "database"=w350, "table"=w351) -> ("输出数组"=w343:string[])  [unwired: 6 in, 1 out]
            n224 = Index Array(array=w348) -> (element=w341:string)  [unwired: 1 in]
            n225 = Index Array(array=w343) -> (element=w342:string)  [unwired: 1 in]
            n226 = control-ref of="自定义数值结束 2"() -> (w357:refnum<vi>)
            n227 = control-ref of="自定义数值起始 2"() -> (w358:refnum<vi>)
            n228 = Fract/Exp String To Number(string=w341) -> (number=w346:dbl)  [unwired: 3 in, 1 out]
            n229 = Fract/Exp String To Number(string=w342) -> (number=w347:dbl)  [unwired: 3 in, 1 out]
            n230 = Bundle By Name(cluster=cluster{"起始范围":string, "截止范围":string} {"起始范围"="2", "截止范围"="5"} ("Single"), "起始范围"=w342, "截止范围"=w341) -> (w345:cluster{"起始范围":string, "截止范围":string})
            n231 = property class="DigNum (严格)"(reference=w357, "Visible"=w356, "Value"=w346) -> ()  [unwired: 1 in, 2 out]
            n232 = property class="DigNum (严格)"(reference=w358, "Visible"=w356, "Value"=w347) -> ()  [unwired: 1 in, 2 out]
            n233 = local write "自定义2single"(w345) -> ()
          }
          frame "Date/Time" {
            n234 = local read "database"() -> (w370:string)
            n235 = property class="Str"(reference=w374, "Visible"=TRUE ("可见")) -> ()  [unwired: 1 in, 2 out]
            n236 = local read "table"() -> (w371:string)
            n237 = call "查询clonm对应的所有内容.vi"("条件"=enum16{"DISTINCT", "MIN", "MAX"}."MAX", "组合框"=w367, "database"=w370, "table"=w371) -> ("输出数组"=w369:string[])  [unwired: 6 in, 1 out]
            n238 = call "查询clonm对应的所有内容.vi"("条件"=enum16{"DISTINCT", "MIN", "MAX"}."MIN", "组合框"=w367, "database"=w370, "table"=w371) -> ("输出数组"=w368:string[])  [unwired: 6 in, 1 out]
            n239 = Index Array(array=w369) -> (element=w362:string)  [unwired: 1 in]
            n240 = Index Array(array=w368) -> (element=w360:string)  [unwired: 1 in]
            n241 = call "格式日期时间字符串.vi"("data[0]"=w362) -> ("日期/时间字符串"=w361:string)  [unwired: 10 in]
            n242 = call "格式日期时间字符串.vi"("data[0]"=w360) -> ("日期/时间字符串"=w359:string)  [unwired: 10 in]
            n243 = control-ref of="自定义起始时间 2"() -> (w376:refnum<vi>)
            n244 = control-ref of="自定义结束时间 2"() -> (w377:refnum<vi>)
            n245 = call "日期字符串格式至时间格式转换(子VI).vi"("data[0]"=w361) -> ("time stamp"=w366:timestamp)  [unwired: 10 in]
            n246 = call "日期字符串格式至时间格式转换(子VI).vi"("data[0]"=w359) -> ("time stamp"=w365:timestamp)  [unwired: 10 in]
            n247 = Bundle By Name(cluster=cluster{"起始范围":string, "截止范围":string} {"起始范围"="2", "截止范围"="5"} ("Single"), "起始范围"=w359, "截止范围"=w361) -> (w364:cluster{"起始范围":string, "截止范围":string})
            n248 = property class="AbsTime (严格)"(reference=w377, "Visible"=TRUE ("可见"), "Value"=w366) -> ()  [unwired: 1 in, 2 out]
            n249 = property class="AbsTime (严格)"(reference=w376, "Visible"=TRUE ("可见"), "Value"=w365) -> ()  [unwired: 1 in, 2 out]
            n250 = local write "自定义2single"(w364) -> ()
          }
        }
      }
      event "清空": Value Change {
        n251 = event-data() -> ()  [unwired: 1 in, 6 out]
        n252 = control-ref of="实时分钟小时数据"() -> (w382:refnum<vi>)
        n253 = control-ref of="组合框 2"() -> (w380:refnum<vi>)
        n254 = control-ref of="组合框"() -> (w381:refnum<vi>)
        n255 = control-ref of="测量模式"() -> (w386:refnum<vi>)
        n256 = control-ref of="自定义 2"() -> (w383:refnum<vi>)
        n257 = control-ref of="自定义"() -> (w384:refnum<vi>)
        n258 = Build Array(w386, w382, w383, w384, w380, w381) -> (w385:refnum<vi>[])
        n259 = for {
          tunnel: w385 -> [w387] mode=indexing
          n260 = invoke class="Ctl" method="Reinit To Default"(reference=w387) -> ()  [unwired: 2 in, 3 out]
        }
      }
      event "确定": Value Change {
        w388 = TRUE
        n261 = event-data() -> ()  [unwired: 1 in, 6 out]
      }
      event "退出": Value Change {
        n262 = event-data() -> ()  [unwired: 1 in, 6 out]
      }
    }
  }
  "确定输出" <- w10
